vi "Read PanelRef.vi"(8 "error in (no error)":errorcluster, 11 "ICD System Tree View in":refnum<class "[V]System Tree View.lvclass">) -> (0 "error out":errorcluster, 2 "PanelRef":refnum<vi>, 3 "ICD System Tree View out":refnum<class "[V]System Tree View.lvclass">)   [LabVIEW 2020]
uses:
  [V]System Tree View.lvclass
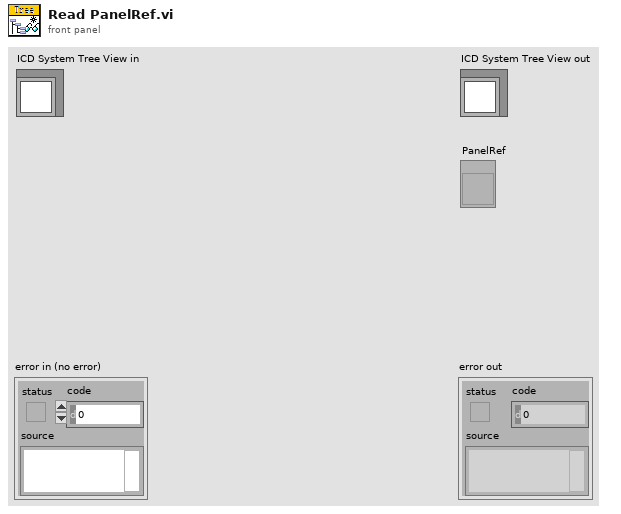
[diagram p1: front panel]
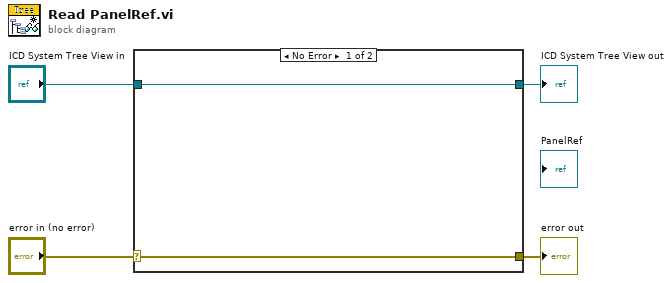
[diagram p0: block diagram]
diagram:
  n1 = case shown="No Error" "error in (no error)" {
    selector: "error in (no error)" -> [w6 w7]
    tunnel: [w6 w7] -> w3
    tunnel: [w5 w8] -> w1
    tunnel: "ICD System Tree View in" -> [w5 w8]
    frame No Error {
    }
    frame Error {
    }
  }
  "error out" <- w3
  "ICD System Tree View out" <- w1
